vi "FA_CreateIfMissing.vi"(8 "Error In":errorcluster) -> (0 "Error Out":errorcluster)   [LabVIEW 2014, in "FA_AgentConfig.lvlib"]
doc: "If FA_Config.xml is not on the system or it does not have all the required config information for FlockAgent to opperate it creates the XML data with default data. The defaults created are as follows. \n\nCloud LookupTime = 1 hour\nDebug = False\nDeviceName = <device serial number> RT, testdevice (Win)\n\nDefault values for x-ni-cloud-id and x-ni-api-key are not created."
uses:
  FA_AgentConfig.lvlib
  FA_LocalStore API/source/VI Source/FA_LocalStore.lvlib
  FA_LocalStore API/source/VI Source/FA_LSSpecialTypes.ctl
  FA_NativeTypes API/source/VI Source/FA_NativeTypes.lvlib
  <resource>/objmgr/nisysapi.rc
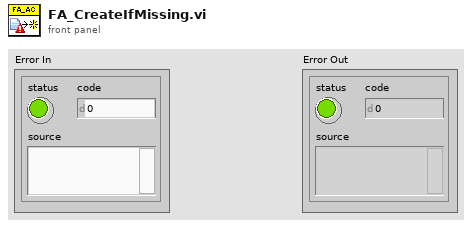
[diagram p1: front panel]
types:
  T1 = typedef "FA_LocalStore.lvlib/FA_LSSpecialTypes.ctl" = string
  T2 = typedef "FA_NativeTypes.lvlib/FA_Config.ctl" = cluster{"Id":string, "Name":T1, "Parameter":cluster{"Name":string, "Value":string}[], "Account":string, "CreateDate":string, "LastModified":string}
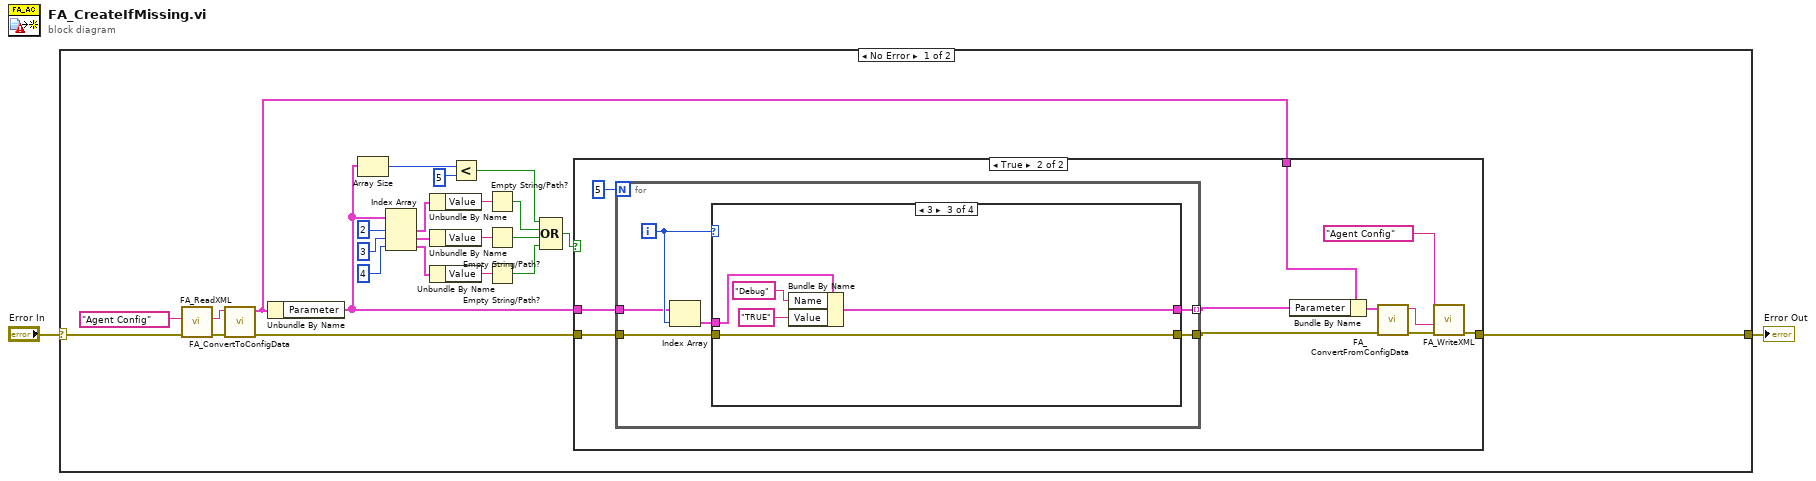
[diagram p0: block diagram]
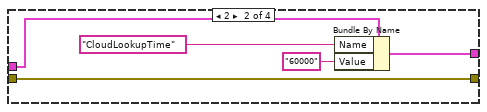
[diagram p4: hidden frame]
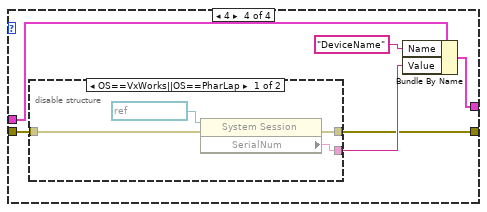
[diagram p5: hidden frame]
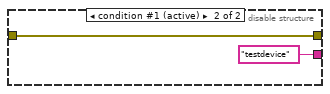
[diagram p6: hidden frame]
diagram:
  n1 = case shown="No Error" "Error In" {
    selector: "Error In" -> [w25 w69]
    tunnel: [w3 w69] -> w1
    frame No Error {
      n2 = call "FA_ReadXML.vi"("Error In"=w25, "Special Type"=T1 "Agent Config") -> ("Error Out"=w24:errorcluster, "XML String"=w23:string)  [unwired: 6 in]
      n3 = call "FA_ConvertToConfigData.vi"("Error In"=w24, "XML String"=w23) -> ("Error Out"=w22:errorcluster, "ConfigData"=w4:T2)  [unwired: 8 in]
      n4 = Unbundle By Name(w4) -> ("Parameter"=w19:cluster{"Name":string, "Value":string}[])
      n5 = Array Size(array=w19) -> (size(s)=w21:i32)
      n6 = Index Array(array=w19, index #1=2 ("index"), index #2=3 ("index"), index #3=4 ("index")) -> (element #1=w15:cluster{"Name":string, "Value":string}, element #2=w14:cluster{"Name":string, "Value":string}, element #3=w13:cluster{"Name":string, "Value":string})
      n7 = Unbundle By Name(w15) -> ("Value"=w12:string)
      n8 = Unbundle By Name(w14) -> ("Value"=w11:string)
      n9 = Unbundle By Name(w13) -> ("Value"=w10:string)
      n10 = Less?(x=w21, y=5) -> (x < y?=w9:bool)
      n11 = Empty String/Path?(string/path=w12) -> (empty?=w8:bool)
      n12 = Empty String/Path?(string/path=w11) -> (empty?=w7:bool)
      n13 = Empty String/Path?(string/path=w10) -> (empty?=w6:bool)
      n14 = Compound Arithmetic op=OR(w9, w8, w7, w6) -> (w5:bool)
      n15 = case shown="True" w5 {
        tunnel: w22 -> [w27 w38]
        tunnel: w19 -> [_ w36]
        tunnel: [w27 w29] -> w3
        tunnel: w4 -> [_ w30]
        frame False {
        }
        frame True {
          n16 = for {
            N: 5 -> [_]
            tunnel: w36 -> [w39]
            tunnel: w38 -> [w44]
            tunnel: [w43] -> w28
            tunnel: [w42] -> w31 mode=indexing
            i -> [w40]
            n17 = Index Array(array=w39, index=w40) -> (element=w41:cluster{"Name":string, "Value":string})
            n18 = case shown="3" w40 {
              tunnel: w41 -> [w45 w51 w56 w62]
              tunnel: w44 -> [w46 w48 w53 w61]
              tunnel: [w46 w48 w53 w58] -> w43
              tunnel: [w45 w47 w52 w57] -> w42
              frame 0, Default {
              }
              frame 2 {
                n19 = Bundle By Name(cluster=w51, "Name"="CloudLookupTime", "Value"="60000") -> (w47:cluster{"Name":string, "Value":string})
              }
              frame 3 {
                n20 = Bundle By Name(cluster=w56, "Name"="Debug", "Value"="TRUE") -> (w52:cluster{"Name":string, "Value":string})
              }
              frame 4 {
                n21 = disable-structure shown="OS==VxWorks||OS==PharLap" {
                  disable-tunnel: w61 -> [w66 w67]
                  disable-tunnel: [w65 "testdevice" ("SerialNum")] -> w60
                  disable-tunnel: [w64 w67] -> w58
                  frame condition #0 {
                    n22 = property class="System Session"(reference=refnum<k21> "localhost" ("System Session"), error in=w66) -> (error out=w64:errorcluster, "SerialNum"=w65:string)  [unwired: 1 out]
                  }
                  frame condition #1 (active) {
                  }
                }
                n23 = Bundle By Name(cluster=w62, "Name"="DeviceName", "Value"=w60) -> (w57:cluster{"Name":string, "Value":string})
              }
            }
          }
          n24 = Bundle By Name(cluster=w30, "Parameter"=w31) -> (w32:T2)
          n25 = call "FA_ConvertFromConfigData.vi"("Error In"=w28, "Config"=w32) -> ("Error Out"=w33:errorcluster, "XML String"=w35:string)  [unwired: 8 in]
          n26 = call "FA_WriteXML.vi"("Error In"=w33, "XML String"=w35, "Special Type"=T1 "Agent Config") -> ("Error Out"=w29:errorcluster)  [unwired: 6 in]
        }
      }
    }
    frame Error {
    }
  }
  "Error Out" <- w1
